vi "CRYPEAQ Loudness Main.vi"(0 "Fl":dbl[](array[numeric])=[20.0, 22.454773997922736, 22.97758714371529, 23.51258021383542, 24.060036879710538, 24.6202474215474, 25.193508881725744, 25.780125222574476, 26.380407487261397, 26.99467396487717, 27.62325035931701, 28.26646996176788, 28.92467382730014, 29.598210956047147, 30.287438477900952, 30.992721842290486, 31.714435011380765, 32.452960658853264, 33.208690372401655, 33.98202486161858, 34.773374170387285, 35.58315789437015, 36.41180540330013, 37.259756068478765, 38.127459496456304, 39.01537576663182, 39.923975675444694, 40.85374098616558, 41.80516468428786, 42.77875123862532, 43.77501686920085, 44.79448982064225, 45.83771064227755, 46.90523247502523, 47.99762134429284, 49.115456460467634, 50.2593305257138, 51.42985004836605, 52.62763566442533, 53.85332246665549, 55.10756034167334, 56.391014313751576, 57.70436489820836, 59.04830846170678, 60.423557591748676, 61.830841474273164, 63.27090628064966, 64.74451556287737, 66.25245065877897, 67.79551110590032, 69.37451506590403, 70.9902997579681, 72.64372190278358, 74.33565817714842, 76.0670056781684, 77.83868239945207, 79.65162771770717, 81.50680289034209, 83.40519156605784, 85.34780030545036, 87.33565911540498, 89.36982199479563, 91.45136749348208, 93.58139928410841, 95.76104674749965, 97.99146557116102, 100.27383836227469, 102.60937527440015, 104.99931464986868, 107.44492367538494, 109.94749905452376, 112.5083676952281, 115.12888741310817, 117.8104476515396, 120.55447021846123, 123.36241003987485, 126.23575593174236, 129.1760313889854, 132.18479539348297, 135.26364324037172, 138.4142073845422, 141.63815830533997, 144.93720539296265, 148.31309785436, 151.76762564113122, 155.30262039792564, 158.91995643433984, 162.62155171801825, 166.4093688923503, 170.2854163162711, 174.251749129759, 178.31047034303583, 182.46373195196514, 186.71373607895154, 191.06273614043988, 195.51303804181413, 200.06700139989707, 204.72704079434857, 209.49562704746577, 214.37528853468135, 219.3686125246637, 224.47824655161554, 229.70689981887307, 235.057344635006, 240.53241788431615, 246.135022530637, 251.86812915653312, 257.73477753839944, 263.73807825806085, 269.881214352571, 276.1674430011124, 282.6000972524956, 289.18258779245804, 295.91840475156465, 302.81111955630627, 309.8643868222997, 317.081946292187, 324.4676248185348, 332.0253383927343, 339.75909422140023, 347.67299285107083, 355.7712303422073, 364.0581004944929, 372.5379971226333, 381.2154163868554, 390.0949591762076, 399.1813335484587, 408.47935722609816, 417.99396015083505, 427.7301870974983, 437.6932003488361, 447.8882824328153, 458.3208389232213, 468.99640130595765, 479.92062991154586, 491.09931691702474, 502.5383894162503, 514.2439125630955, 526.2220927869496, 538.4792810835186, 551.0219763824239, 563.8568289927026, 576.9906441289077, 590.4303855198066, 604.1831790999819, 618.2563167885307, 632.6572603549645, 647.3936453762086, 662.4732852843022, 677.9041755094981, 693.6944977199626, 709.8526241591744, 726.387122085026, 743.3067583130218, 760.6205038636788, 778.3375387195264, 796.4672566926057, 815.0192704046698, 834.0034163843833, 853.429760282622, 873.3086022095733, 893.6504821954353, 914.4661857797167, 935.7667497292374, 957.5634678900275, 979.8678971760271, 1002.6918636957867, 1026.0474690237668, 1049.9470966162373, 1074.4034183769784, 1099.429401376779, 1125.0383147279376, 1151.2437366204622, 1178.059561520769, 1205.5000075390842, 1233.5796239681415, 1262.3132989970838, 1291.716267605563, 1321.8041196417378, 1352.592808087576, 1384.0986575181541, 1416.3383727566554, 1449.329047731571, 1483.0881745401007, 1517.6336527227509, 1552.983798754135, 1589.1573557540758, 1626.173503426001, 1664.0518682259462, 1702.8125337688543, 1742.4760514771751, 1783.0634514774647, 1824.596253750986, 1867.0964795436084, 1910.5866630422083, 1955.0898633219676, 2000.629676573275, 2047.2302486121253, 2094.916287683119, 2143.7130775595638, 2193.6464909496717, 2244.7430032145617, 2297.0297064054575, 2350.534323628789, 2405.2852237450925, 2461.3114364103076, 2518.642667468382, 2577.309314700866, 2637.342483944817, 2698.774005585298, 2761.636451432274, 2825.9631519907193, 2891.788214132709, 2959.1465391814268, 3028.073841416658, 3098.6066670100945, 3170.7824134035327, 3244.6393491370727, 3320.21663413942, 3397.554340491384, 3476.69347367248, 3557.675994302525, 3640.544840389543, 3725.3439500966592, 3812.118285038006, 3900.9138541182183, 3991.777737927235, 4084.7581137026004, 4179.904280874161, 4277.266687202766, 4376.896955528673, 4478.84791114254, 4583.173609794229, 4689.9293663536055, 4799.17178413954, 4910.958784931605, 5025.349639680679, 5142.40499993584, 5262.186930001873, 5384.7589398471655, 5510.186018777306, 5638.534669893191, 5769.872945352114, 5904.270482449578, 6041.798540542085, 6182.530038829943, 6326.539595019659, 6473.903564887547, 6624.700082764322, 6779.009102963305, 6936.912442172715, 7098.493822836377, 7263.838917544618, 7433.0353944582685, 7606.172963792461, 7783.34342538143, 7964.640717352117, 8150.16096593186, 8340.002536415303, 8534.266085318994, 8733.05461375138, 8936.473522024511, 9144.630665539245, 9357.636411971636, 9575.60369979094, 9798.648098141424] format="%#.6g", 1 "Fs":dbl=44100.0, 3 "NF":dbl=2048.0, 5 "Fc":dbl[](array[numeric]), 7 "Fu":dbl[](array[numeric])=[22.454773997922736, 22.97758714371529, 23.51258021383542, 24.060036879710538, 24.6202474215474, 25.193508881725744, 25.780125222574476, 26.380407487261397, 26.99467396487717, 27.62325035931701, 28.26646996176788, 28.92467382730014, 29.598210956047147, 30.287438477900952, 30.992721842290486, 31.714435011380765, 32.452960658853264, 33.208690372401655, 33.98202486161858, 34.773374170387285, 35.58315789437015, 36.41180540330013, 37.259756068478765, 38.127459496456304, 39.01537576663182, 39.923975675444694, 40.85374098616558, 41.80516468428786, 42.77875123862532, 43.77501686920085, 44.79448982064225, 45.83771064227755, 46.90523247502523, 47.99762134429284, 49.115456460467634, 50.2593305257138, 51.42985004836605, 52.62763566442533, 53.85332246665549, 55.10756034167334, 56.391014313751576, 57.70436489820836, 59.04830846170678, 60.423557591748676, 61.830841474273164, 63.27090628064966, 64.74451556287737, 66.25245065877897, 67.79551110590032, 69.37451506590403, 70.9902997579681, 72.64372190278358, 74.33565817714842, 76.0670056781684, 77.83868239945207, 79.65162771770717, 81.50680289034209, 83.40519156605784, 85.34780030545036, 87.33565911540498, 89.36982199479563, 91.45136749348208, 93.58139928410841, 95.76104674749965, 97.99146557116102, 100.27383836227469, 102.60937527440015, 104.99931464986868, 107.44492367538494, 109.94749905452376, 112.5083676952281, 115.12888741310817, 117.8104476515396, 120.55447021846123, 123.36241003987485, 126.23575593174236, 129.1760313889854, 132.18479539348297, 135.26364324037172, 138.4142073845422, 141.63815830533997, 144.93720539296265, 148.31309785436, 151.76762564113122, 155.30262039792564, 158.91995643433984, 162.62155171801825, 166.4093688923503, 170.2854163162711, 174.251749129759, 178.31047034303583, 182.46373195196514, 186.71373607895154, 191.06273614043988, 195.51303804181413, 200.06700139989707, 204.72704079434857, 209.49562704746577, 214.37528853468135, 219.3686125246637, 224.47824655161554, 229.70689981887307, 235.057344635006, 240.53241788431615, 246.135022530637, 251.86812915653312, 257.73477753839944, 263.73807825806085, 269.881214352571, 276.1674430011124, 282.6000972524956, 289.18258779245804, 295.91840475156465, 302.81111955630627, 309.8643868222997, 317.081946292187, 324.4676248185348, 332.0253383927343, 339.75909422140023, 347.67299285107083, 355.7712303422073, 364.0581004944929, 372.5379971226333, 381.2154163868554, 390.0949591762076, 399.1813335484587, 408.47935722609816, 417.99396015083505, 427.7301870974983, 437.6932003488361, 447.8882824328153, 458.3208389232213, 468.99640130595765, 479.92062991154586, 491.09931691702474, 502.5383894162503, 514.2439125630955, 526.2220927869496, 538.4792810835186, 551.0219763824239, 563.8568289927026, 576.9906441289077, 590.4303855198066, 604.1831790999819, 618.2563167885307, 632.6572603549645, 647.3936453762086, 662.4732852843022, 677.9041755094981, 693.6944977199626, 709.8526241591744, 726.387122085026, 743.3067583130218, 760.6205038636788, 778.3375387195264, 796.4672566926057, 815.0192704046698, 834.0034163843833, 853.429760282622, 873.3086022095733, 893.6504821954353, 914.4661857797167, 935.7667497292374, 957.5634678900275, 979.8678971760271, 1002.6918636957867, 1026.0474690237668, 1049.9470966162373, 1074.4034183769784, 1099.429401376779, 1125.0383147279376, 1151.2437366204622, 1178.059561520769, 1205.5000075390842, 1233.5796239681415, 1262.3132989970838, 1291.716267605563, 1321.8041196417378, 1352.592808087576, 1384.0986575181541, 1416.3383727566554, 1449.329047731571, 1483.0881745401007, 1517.6336527227509, 1552.983798754135, 1589.1573557540758, 1626.173503426001, 1664.0518682259462, 1702.8125337688543, 1742.4760514771751, 1783.0634514774647, 1824.596253750986, 1867.0964795436084, 1910.5866630422083, 1955.0898633219676, 2000.629676573275, 2047.2302486121253, 2094.916287683119, 2143.7130775595638, 2193.6464909496717, 2244.7430032145617, 2297.0297064054575, 2350.534323628789, 2405.2852237450925, 2461.3114364103076, 2518.642667468382, 2577.309314700866, 2637.342483944817, 2698.774005585298, 2761.636451432274, 2825.9631519907193, 2891.788214132709, 2959.1465391814268, 3028.073841416658, 3098.6066670100945, 3170.7824134035327, 3244.6393491370727, 3320.21663413942, 3397.554340491384, 3476.69347367248, 3557.675994302525, 3640.544840389543, 3725.3439500966592, 3812.118285038006, 3900.9138541182183, 3991.777737927235, 4084.7581137026004, 4179.904280874161, 4277.266687202766, 4376.896955528673, 4478.84791114254, 4583.173609794229, 4689.9293663536055, 4799.17178413954, 4910.958784931605, 5025.349639680679, 5142.40499993584, 5262.186930001873, 5384.7589398471655, 5510.186018777306, 5638.534669893191, 5769.872945352114, 5904.270482449578, 6041.798540542085, 6182.530038829943, 6326.539595019659, 6473.903564887547, 6624.700082764322, 6779.009102963305, 6936.912442172715, 7098.493822836377, 7263.838917544618, 7433.0353944582685, 7606.172963792461, 7783.34342538143, 7964.640717352117, 8150.16096593186, 8340.002536415303, 8534.266085318994, 8733.05461375138, 8936.473522024511, 9144.630665539245, 9357.636411971636, 9575.60369979094, 9798.648098141424, 18000.0] format="%#.6g", 11 "Internal Noise":dbl[](array[numeric]), 12 "X2R":dbl[](array[numeric]), 14 "X2T":dbl[](array[numeric])) -> (8 "Response Ntotal":dbl, 10 "Stimulus Ntotal":dbl, 13 "fc":dbl[](array[numeric]), 15 "NL":dbl)   [LabVIEW 2013]
panel:
  out "Test":cluster{"Fc":dbl[], "Es":dbl[]}[](graph)
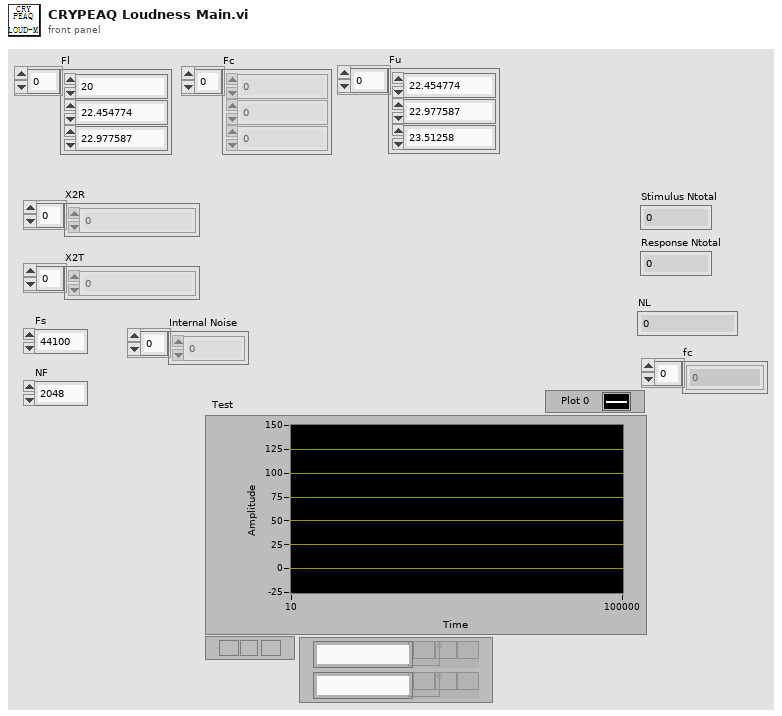
[diagram p1: front panel]
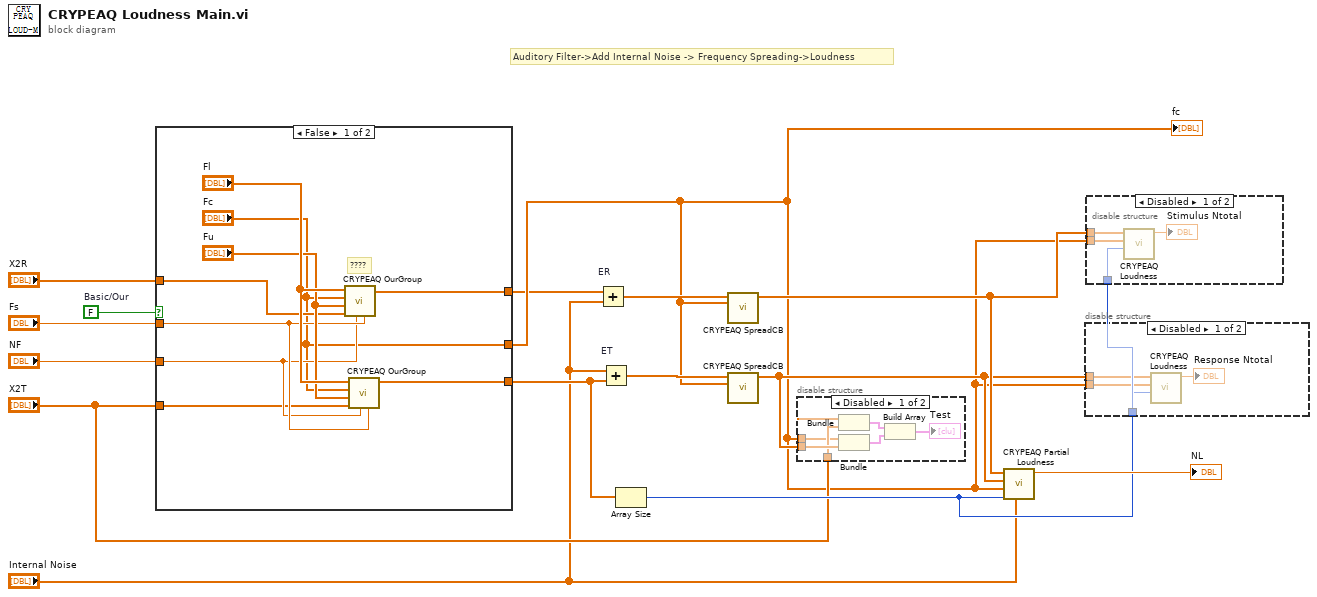
[diagram p0: block diagram]
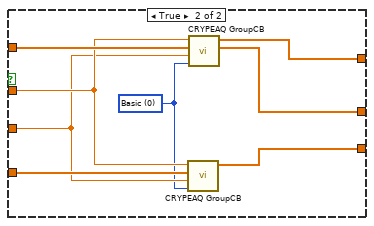
[diagram p5: hidden frame]
diagram:
  w7 = FALSE  # Basic/Our
  # "Auditory Filter->Add Internal Noise -> Frequency Spreading->Loudness"
  n1 = case shown="False" w7 {
    tunnel: [w24 w25] -> w2
    tunnel: "Fs" -> [w21 w29]
    tunnel: "NF" -> [w20 w28]
    tunnel: [w19 w26] -> w3
    tunnel: "X2R" -> [w18 w31]
    tunnel: ["Fc" w32] -> w4
    tunnel: "X2T" -> [w17 w30]
    frame False {
      # "????"
      n2 = call "CRYPEAQ OurGroup.vi"("Fs"=w21, "NF"=w20, "E"=w18, "Fu"="Fu", "Fc"="Fc", "Fl"="Fl") -> ("Grouped E"=w24:dbl[])  [unwired: 5 in]
      n3 = call "CRYPEAQ OurGroup.vi"("Fs"=w21, "NF"=w20, "E"=w17, "Fu"="Fu", "Fc"="Fc", "Fl"="Fl") -> ("Grouped E"=w19:dbl[])  [unwired: 5 in]
    }
    frame True {
      w27 = u16 0 items=["Basic", "Advance", "My"] ("Version")
      n4 = call "CRYPEAQ GroupCB.vi"("Version"=w27, "NF"=w28, "X2"=w30, "Fs"=w29) -> ("Eb"=w26:dbl[])  [unwired: 5 in, 2 out]
      n5 = call "CRYPEAQ GroupCB.vi"("Version"=w27, "NF"=w28, "X2"=w31, "Fs"=w29) -> ("fc"=w32:dbl[], "Eb"=w25:dbl[])  [unwired: 5 in, 1 out]
    }
  }
  "fc" <- w4
  n6 = Add "ER"(x=w2, y="Internal Noise") -> (x+y=w5:dbl[])
  n7 = Add "ET"(x="Internal Noise", y=w3) -> (x+y=w6:dbl[])
  n8 = Array Size(array=w3) -> (size(s)=w10:i32)
  n9 = call "CRYPEAQ SpreadCB.vi"("Center Frequency"=w4, "E"=w5) -> ("Es"=w13:dbl[])  [unwired: 8 in, 1 out]
  n10 = call "CRYPEAQ SpreadCB.vi"("Center Frequency"=w4, "E"=w6) -> ("Es"=w12:dbl[])  [unwired: 8 in, 1 out]
  n11 = disable-structure shown="Disabled" {
    disable-tunnel: w12 -> [w38 _]
    disable-tunnel: "X2T" -> [w34 _]
    disable-tunnel: w4 -> [w33 _]
    frame Disabled {
      n12 = Bundle("fc"=w33, "X2T"=w34) -> (w36:cluster{"fc":dbl[], "X2T":dbl[]})  [unwired: 1 in]
      n13 = Bundle("fc"=w33, "Es"=w38) -> (w37:cluster{"fc":dbl[], "Es":dbl[]})  [unwired: 1 in]
      n14 = Build Array(w36, w37) -> (→"Test":cluster{"fc":dbl[], "Es":dbl[]}[])
    }
    frame Enabled {
    }
  }
  n15 = call "CRYPEAQ Partial Loudness.vi"("Internal Noise"="Internal Noise", "Nc"=w10, "fc"=w4, "EPT"=w12, "EPR"=w13) -> ("NL"=→"NL":dbl)  [unwired: 6 in]
  n16 = disable-structure shown="Disabled" {
    disable-tunnel: w12 -> [w42 _]
    disable-tunnel: w10 -> [w41 _]
    disable-tunnel: w4 -> [w40 _]
    frame Disabled {
      n17 = call "CRYPEAQ Loudness.vi"("Nc"=w41, "fc"=w40, "Ehs"=w42) -> ("Ntotal"=→"Response Ntotal":dbl)  [unwired: 7 in]
    }
    frame Enabled {
    }
  }
  n18 = disable-structure shown="Disabled" {
    disable-tunnel: w13 -> [w45 _]
    disable-tunnel: w10 -> [w44 _]
    disable-tunnel: w4 -> [w43 _]
    frame Disabled {
      n19 = call "CRYPEAQ Loudness.vi"("Nc"=w44, "fc"=w43, "Ehs"=w45) -> ("Ntotal"=→"Stimulus Ntotal":dbl)  [unwired: 7 in]
    }
    frame Enabled {
    }
  }
